vi "Get Name.vi"(8 "error in (no error)":errorcluster, 11 "Form Configuration in":refnum<class "Form Configuration.lvclass">) -> (0 "error out":errorcluster, 2 "Form ID":T1, 3 "Form Configuration out":refnum<class "Form Configuration.lvclass">)   [LabVIEW 2020, in "Form Configuration.lvlib" / "Form Configuration.lvclass"]
uses:
  Form Configuration.lvclass
  Form ID.ctl
  Form Configuration.lvclass/Form Configuration.ctl
  Form Server Interfaces.lvlib
  <vilib>/MGI/Panel Manager/Panel/Panel/Panel.lvclass
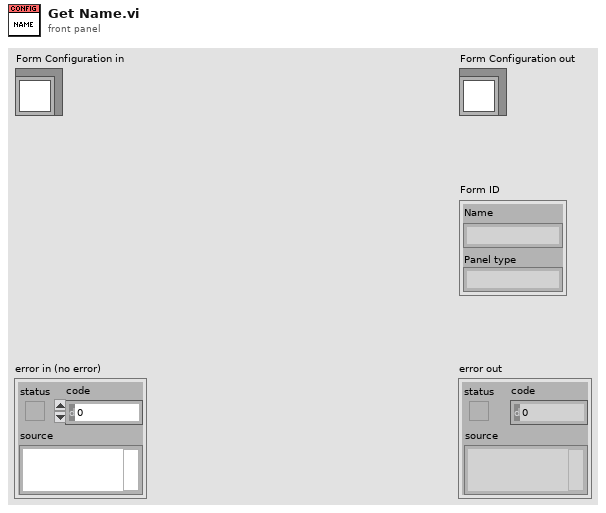
[diagram p1: front panel]
types:
  T1 = typedef "Form Server Interfaces.lvlib/Form ID.ctl" = cluster{"Name":string, "Panel type":string}
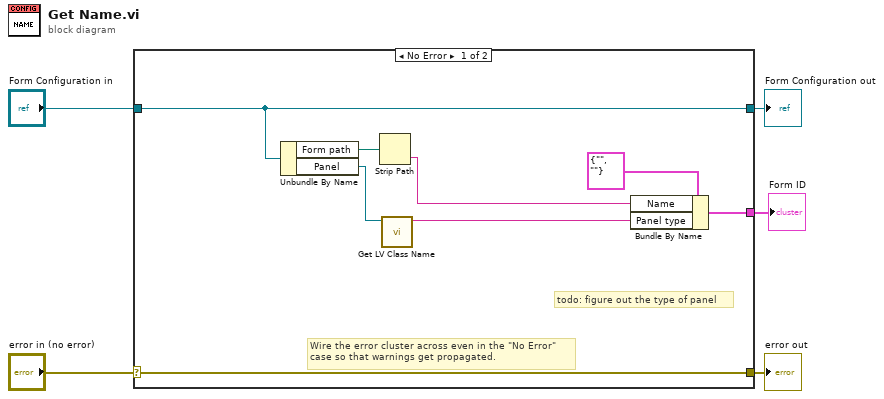
[diagram p0: block diagram]
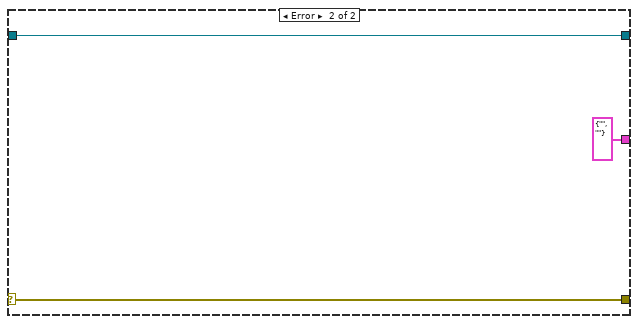
[diagram p2: hidden frame]
diagram:
  n1 = case shown="No Error" "error in (no error)" {
    selector: "error in (no error)" -> [w13 w16]
    tunnel: [w13 w16] -> w4
    tunnel: [w12 w15] -> w2
    tunnel: "Form Configuration in" -> [w12 w15]
    tunnel: [w9 T1 {"Name"="", "Panel type"=""} ("Form ID")] -> w1
    frame No Error {
      # "todo: figure out the type of panel"
      # "Wire the error cluster across even in the \"No Error\"\ncase so that warnings get propagated."
      n2 = Unbundle By Name(w12) -> ("Form path"=w11:path, "Panel"=w7:refnum<class "Panel.lvclass">)
      n3 = Strip Path(path=w11) -> (name=w8:string)  [unwired: 1 out]
      n4 = call <vilib>:"Get LV Class Name.vi"("object"=w7) -> ("class name"=w6:string)  [unwired: 9 in, 1 out]
      n5 = Bundle By Name(cluster=T1 {"Name"="", "Panel type"=""} ("Form ID"), "Name"=w8, "Panel type"=w6) -> (w9:T1)
    }
    frame Error {
    }
  }
  "error out" <- w4
  "Form Configuration out" <- w2
  "Form ID" <- w1
